vi "Adam_Ch_Input_Output.vi"(0 "Ch names":string[](array[string]), 1 "Previous Scan Value":dbl format="%.2f", 3 "Duty No":u16 format="%016b", 5 "Ch Description":T1={"Ch Name"="", "Type"="", "Function"=enum."Analogue Input", "Ch State"=enum."On", "Calibration type"="", "A"=0.0, "B"=0.0, "C"=0.0, "D"=0.0, "Comments"="", "Address"={"Main"=0, "Ch."=0, "Sub"=0, "Port Name"=""}, "String"="", "Duty"=65535} {"Duty" format="%016b"; "D" format="%#_5g"; "C" format="%#_5g"; "B" format="%#_5g"; "A" format="%#_5g"}, 9 "Scan Period":dbl format="%.2f", 11 "Ch values":dbl[](array[numeric]) format="%.2f", 12 "Value to Output":dbl format="%.2f", 13 "Current Time (sec)":dbl format="%.1f", 14 "Simulate":bool) -> (4 "Calibrated units":dbl format="%_3g", 6 "Good Module":string, 8 "chTime(s)":dbl format="%#_3ps", 10 "Error Row":string[](array[string]), 15 "Scan comment":string)   [LabVIEW 2021]
uses:
  ADAM Client/Sub VIs/ADAM Controls/Ch_description_ADAM.ctl
  ADAM Client/Sub VIs/ADAM Controls/Module_type_ADAM.ctl
  ADAM Client/Sub VIs/ADAM Controls/Function_ADAM.ctl
  ADAM Client/Sub VIs/ADAM Controls/Channel_State.ctl
  ADAM Client/Sub VIs/ADAM Controls/Calib_type_ADAM.ctl
  ADAM Client/Sub VIs/ADAM Controls/Address.ctl
  ADAM_Global.vi
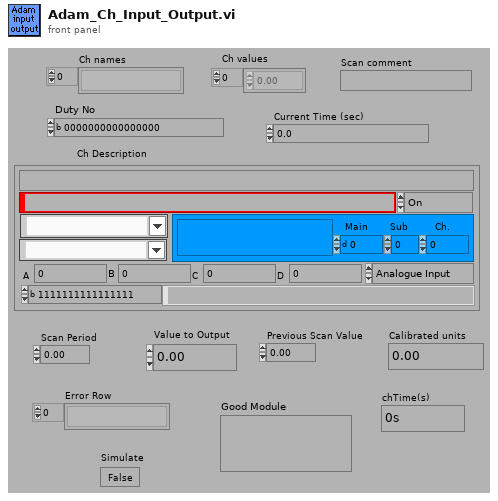
[diagram p1: front panel]
types:
  T1 = typedef "Ch_description_ADAM.ctl" = cluster{"Ch Name":string, "Type":T2, "Function":T3, "Ch State":T4, "Calibration type":T5, "A":dbl, "B":dbl, "C":dbl, "D":dbl, "Comments":string, "Address":T6, "String":string, "Duty":u16}
  T2 = typedef "Module_type_ADAM.ctl" = string
  T3 = typedef "Function_ADAM.ctl" = enum16{"Analogue Input", "Digital Input", "Event counter", "Event rate", "Analogue Output", "Digital Output", "Relay Output"}
  T4 = typedef "Channel_State.ctl" = enum16{"On", "Off", "Always On", "Always Off"}
  T5 = typedef "Calib_type_ADAM.ctl" = string
  T6 = typedef "Address.ctl" = cluster{"Main":i32, "Ch.":i32, "Sub":i32, "Port Name":string}
  T7 = enum16{"On", "Off", "Always On", "Always Off", "Delete"}
  T8 = cluster{"Channel Names":string[], "Last Updated":dbl[]}
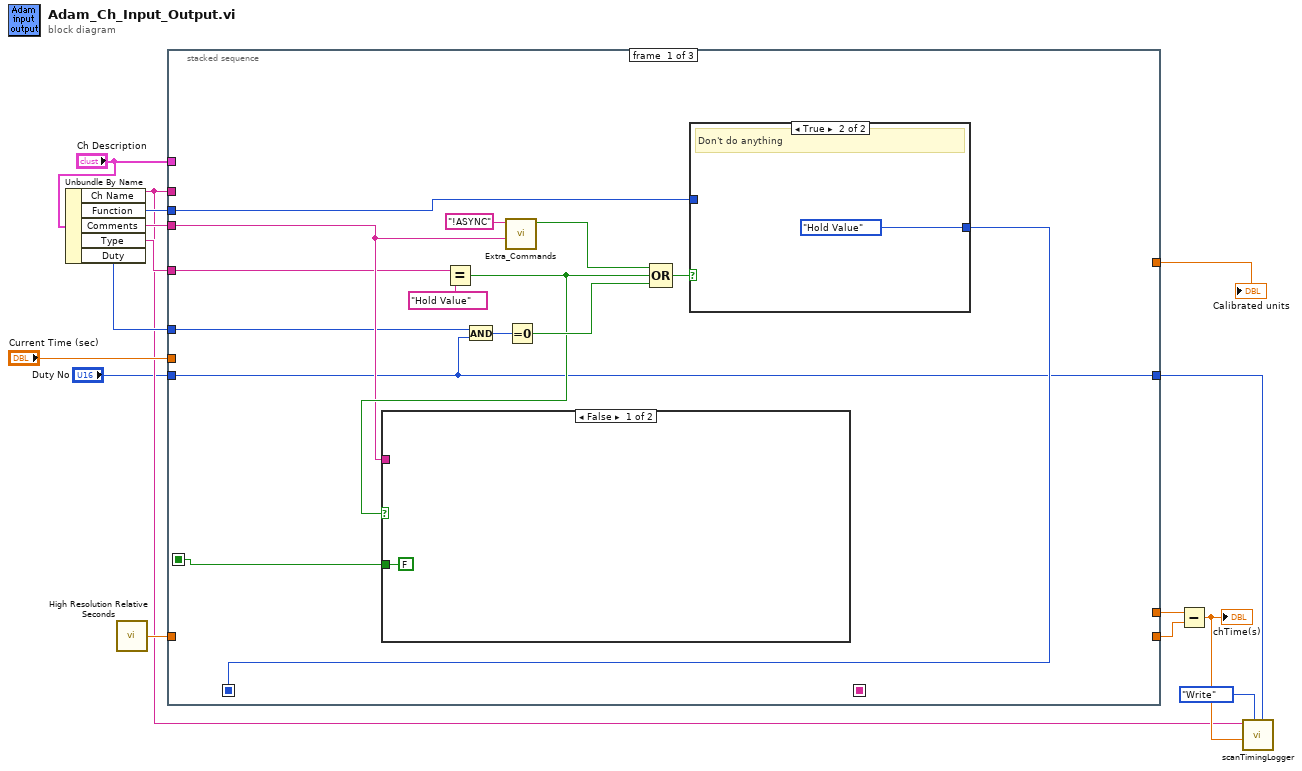
[diagram p0: block diagram]
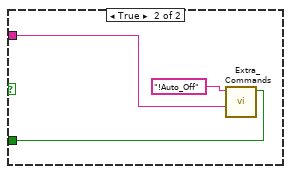
[diagram p2: hidden frame]
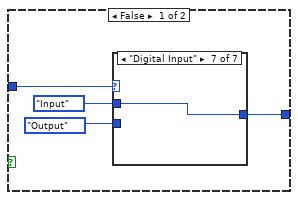
[diagram p3: hidden frame]
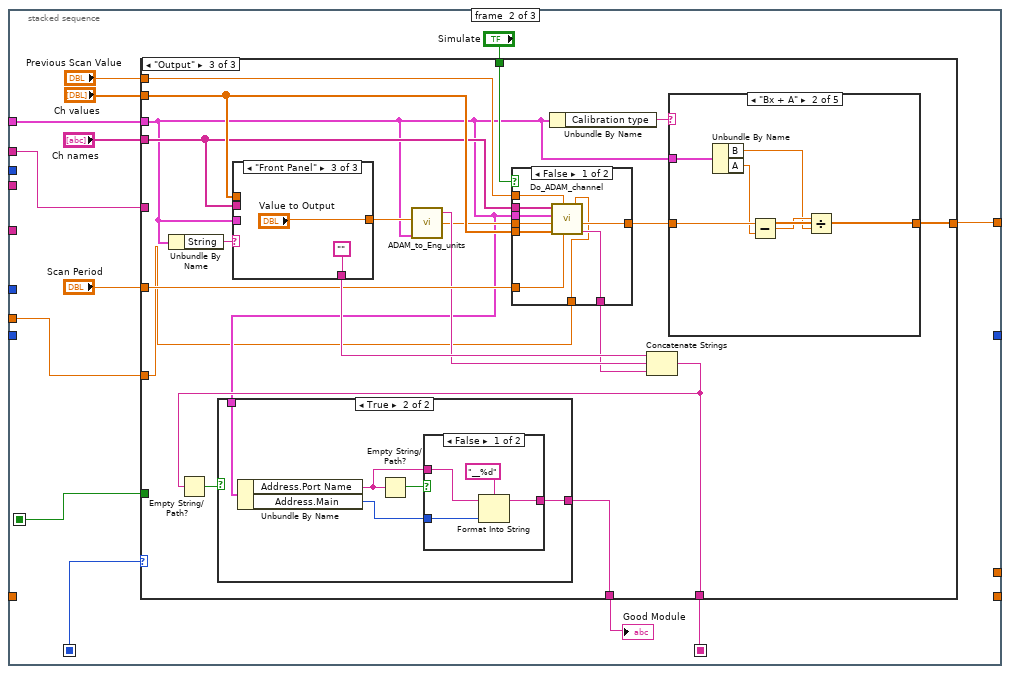
[diagram p10: hidden frame]
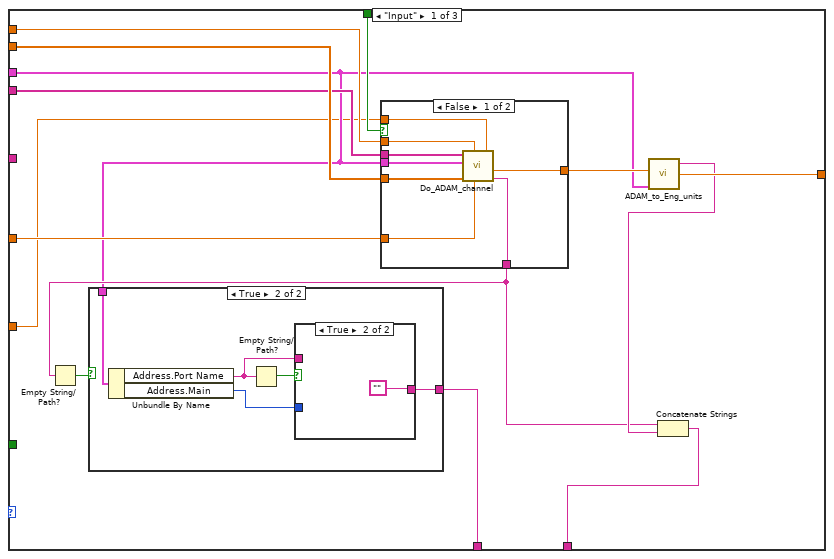
[diagram p11: hidden frame]
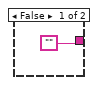
[diagram p12: hidden frame]
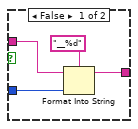
[diagram p13: hidden frame]
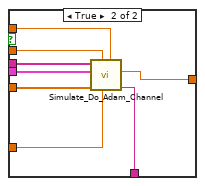
[diagram p14: hidden frame]
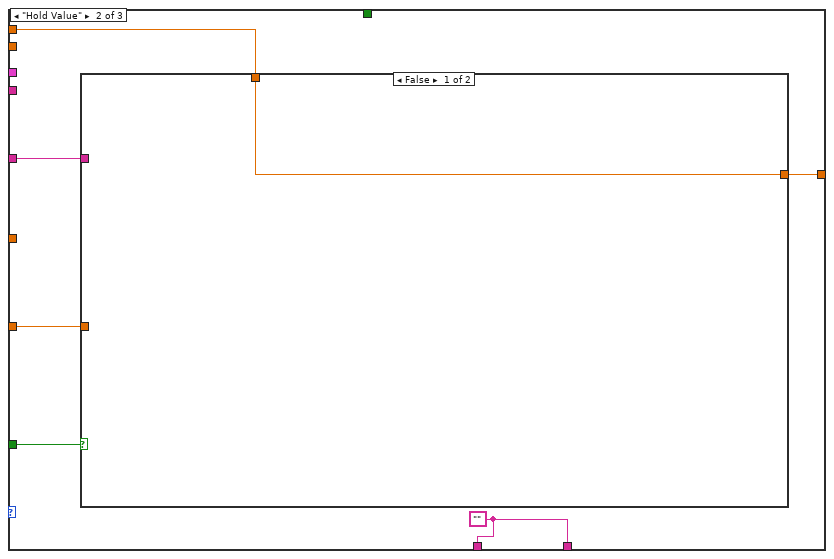
[diagram p15: hidden frame]
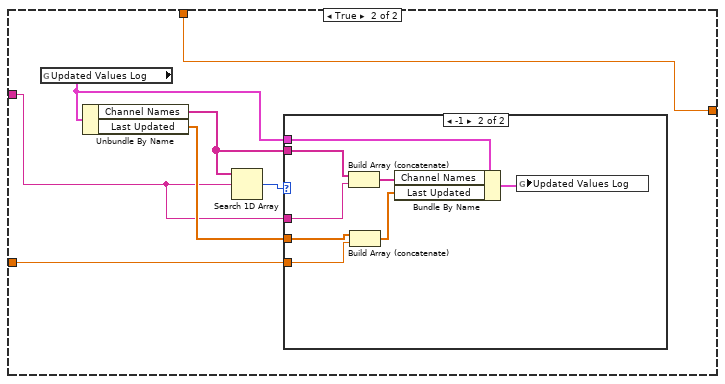
[diagram p16: hidden frame]
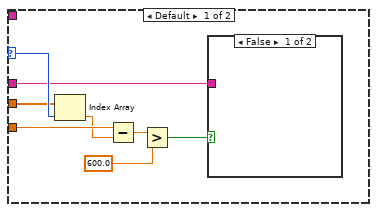
[diagram p17: hidden frame]
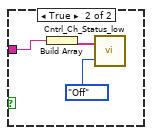
[diagram p18: hidden frame]
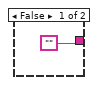
[diagram p19: hidden frame]
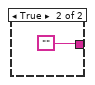
[diagram p20: hidden frame]
diagram:
  n1 = Unbundle By Name("Ch Description") -> ("Ch Name"=w4:string, "Function"=w12:T3, "Comments"=w11:string, "Type"=w10:T2, "Duty"=w9:u16)
  n2 = call <vilib>:"High Resolution Relative Seconds.vi"() -> ("relative seconds"=w6:dbl)
  n3 = stacked-sequence {
    seq-local: [w28 _ _] -> [_ w54 _]
    seq-local: [_ w53 _] -> [_ _ w225]
    seq-local: [w21 _ _] -> [_ w48 _]
    tunnel: "Ch Description" -> [_ w56 w224]
    tunnel: [_ w50 _] -> w14
    tunnel: "Current Time (sec)" -> [_ w47 _]
    tunnel: w12 -> [w20 _ _]
    tunnel: w11 -> [w19 _ _]
    tunnel: w10 -> [w18 _ _]
    tunnel: w9 -> [w17 _ _]
    tunnel: w4 -> [_ w46 _]
    tunnel: [_ _ w222] -> w8
    tunnel: [_ _ w221] -> w7
    tunnel: w6 -> [_ _ w221]
    tunnel: [w16 _ _] -> w2
    tunnel: "Duty No" -> [w16 _ _]
    frame #0 {
      n4 = Equal?(x=w18, y=T2 "Hold Value" ("Type")) -> (x = y?=w22:bool)
      n5 = case shown="False" w22 {
        tunnel: w19 -> [_ w33]
        tunnel: [FALSE ("Command Found") w31] -> w21
        frame False {
        }
        frame True {
          n6 = call "Extra_Commands.vi"("String to Search"=w33, "Command"="!Auto_Off" ("String to match")) -> ("Command Found"=w31:bool)  [unwired: 1 in, 4 out]
        }
      }
      n7 = And(x=w17, y=w16) -> (x .and. y?=w25:u16)
      n8 = call "Extra_Commands.vi"("String to Search"=w19, "Command"="!ASYNC" ("String to match")) -> ("Command Found"=w26:bool)  [unwired: 1 in, 4 out]
      n9 = Equal To 0?(x=w25) -> (x = 0?=w24:bool)
      n10 = Compound Arithmetic op=OR(w26, w22, w24) -> (w23:bool)
      n11 = case shown="True" w23 {
        tunnel: w20 -> [w35 _]
        tunnel: [w34 enum16{"Input", "Output", "Hold Value"}."Hold Value"] -> w28
        frame False {
          n12 = case shown="\"Digital Input\"" w35 {
            tunnel: [w38 w39 w40 w41 w42 w43 w44] -> w34
            tunnel: enum16{"Input", "Output", "Hold Value"}."Input" -> [w38 w39 w40 _ _ _ w44]
            tunnel: enum16{"Input", "Output", "Hold Value"}."Output" -> [_ _ _ w41 w42 w43 _]
            frame "Analogue Input" {
            }
            frame "Event counter" {
            }
            frame "Event rate" {
            }
            frame "Analogue Output" {
            }
            frame "Digital Output" {
            }
            frame "Relay Output" {
            }
            frame "Digital Input" {
            }
          }
        }
        frame True {
          # "Don't do anything"
        }
      }
    }
    frame #1 {
      n13 = case shown="\"Output\"" w54 {
        tunnel: [w72 w103 w140] -> w50
        tunnel: "Scan Period" -> [w68 _ w145]
        tunnel: "Ch values" -> [w70 _ w151]
        tunnel: "Ch names" -> [w69 _ w150]
        tunnel: [w65 w100 w136] -> w53
        tunnel: w56 -> [w61 _ w134]
        tunnel: "Previous Scan Value" -> [w67 w104 w148]
        tunnel: "Simulate" -> [w64 _ w142]
        tunnel: [w60 w100 w135] -> w49
        tunnel: w48 -> [_ w105 _]
        tunnel: w47 -> [w59 w101 w133]
        tunnel: w46 -> [_ w102 _]
        frame "Input" {
          n14 = case shown="False" w64 {
            tunnel: [w91 w99] -> w71
            tunnel: w70 -> [w90 w98]
            tunnel: w69 -> [w89 w97]
            tunnel: w61 -> [w85 w96]
            tunnel: w68 -> [w88 w95]
            tunnel: w67 -> [w87 w94]
            tunnel: [w86 w93] -> w62
            tunnel: w59 -> [w84 w92]
            frame False {
              n15 = call "Do_ADAM_channel.vi"("Current Time (sec)"=w84, "Scan Period"=w88, "Previous Scan Value"=w87, "Present scan array"=w90, "Ch Description"=w85, "Ch names"=w89) -> ("Scan comment"=w86:string, "Output"=w91:dbl)  [unwired: 1 in, 1 out]
            }
            frame True {
              n16 = call "Simulate_Do_Adam_Channel.vi"("Current Time (sec)"=w92, "Scan Period"=w95, "Previuos Scan Value"=w94, "Ch values"=w98, "Ch Discription"=w96, "Ch names"=w97) -> ("Scan comment"=w93:string, "Calibrated units"=w99:dbl)  [unwired: 3 in]
            }
          }
          n17 = Empty String/Path?(string/path=w62) -> (empty?=w63:bool)
          n18 = case shown="True" w63 {
            tunnel: w61 -> [_ w75]
            tunnel: ["" w74] -> w60
            frame False {
            }
            frame True {
              n19 = Unbundle By Name(w75) -> ("Address.Port Name"=w77:string, "Address.Main"=w76:i32)
              n20 = Empty String/Path?(string/path=w77) -> (empty?=w78:bool)
              n21 = case shown="True" w78 {
                tunnel: w77 -> [w82 _]
                tunnel: w76 -> [w81 _]
                tunnel: [w79 ""] -> w74
                frame False {
                  n22 = Format Into String(format string="__%d", initial string=w82, w81) -> (resulting string=w79:string)  [unwired: 1 in, 1 out]
                }
                frame True {
                }
              }
            }
          }
          n23 = call "ADAM_to_Eng_units.vi"("Ch Description"=w61, "Raw"=w71) -> ("Calibrated units"=w72:dbl, "Comments"=w66:string)  [unwired: 1 in, 2 out]
          n24 = Concatenate Strings(w62, w66) -> (w65:string)
        }
        frame "Hold Value" {
          w100 = ""
          n25 = case shown="False" w105 {
            tunnel: w104 -> [w106 w110]
            tunnel: [w106 w110] -> w103
            tunnel: w102 -> [_ w107]
            tunnel: w101 -> [_ w111]
            frame False {
            }
            frame True {
              n26 = global read "ADAM_Global.vi" "Updated Values Log"() -> (w109:T8)
              n27 = Unbundle By Name(w109) -> ("Channel Names"=w108:string[], "Last Updated"=w112:dbl[])
              n28 = Search 1D Array(1D array=w108, element=w107) -> (index of element=w113:i32)  [unwired: 1 out]
              n29 = case shown="-1" w113 {
                selector: w113 -> [w121 _]
                tunnel: w112 -> [w120 w128]
                tunnel: w111 -> [w119 w127]
                tunnel: w109 -> [_ w132]
                tunnel: w108 -> [_ w131]
                tunnel: w107 -> [w114 w129]
                frame Default {
                  n30 = Index Array(array=w120, index=w121) -> (element=w118:dbl)
                  n31 = Subtract(x=w119, y=w118) -> (x-y=w117:dbl)
                  n32 = Greater?(x=w117, y=600.0) -> (0:w115:bool)
                  n33 = case shown="False" w115 {
                    tunnel: w114 -> [_ w122]
                    frame False {
                    }
                    frame True {
                      n34 = Build Array(w122) -> (w123:string[])
                      n35 = call "Cntrl_Ch_Status_low.vi"("Mode"=T7."Off", "Channel names"=w123) -> ()  [unwired: 1 out]
                    }
                  }
                }
                frame -1 {
                  n36 = Build Array (concatenate)(w131, w129) -> (w130:string[])
                  n37 = Build Array (concatenate)(w128, w127) -> (w126:dbl[])
                  n38 = Bundle By Name(cluster=w132, "Channel Names"=w130, "Last Updated"=w126) -> (w125:T8)
                  n39 = global write "ADAM_Global.vi" "Updated Values Log"(w125) -> ()
                }
              }
            }
          }
        }
        frame "Output" {
          n40 = Unbundle By Name(w134) -> ("String"=w147:string)
          n41 = case shown="\"Front Panel\"" w147 {
            selector: w147 -> [w211 _ _]
            tunnel: w134 -> [_ w218 _]
            tunnel: w151 -> [w215 _ _]
            tunnel: w150 -> [w214 _ _]
            tunnel: [w213 "" ""] -> w149
            tunnel: [w212 w216 "Value to Output"] -> w146
            frame "Other", Default {
              n42 = call "Read_value_of_earlier_Ch.vi"("Desired Ch to Read"=w211, "Ch names"=w214, "Present scan array"=w215) -> ("Value"=w212:dbl, "Scan comment"=w213:string)  [unwired: 1 in]
            }
            frame "Read A" {
              n43 = Unbundle By Name(w218) -> ("A"=w216:dbl)
            }
            frame "Front Panel" {
            }
          }
          n44 = call "ADAM_to_Eng_units.vi"("Ch Description"=w134, "Raw"=w146) -> ("Calibrated units"=w143:dbl, "Comments"=w144:string)  [unwired: 1 in, 2 out]
          n45 = case shown="False" w142 {
            tunnel: w151 -> [w201 w210]
            tunnel: w150 -> [w200 w209]
            tunnel: [w199 w208] -> w139
            tunnel: w148 -> [w198 w207]
            tunnel: [w197 w206] -> w138
            tunnel: w145 -> [w196 w205]
            tunnel: w134 -> [w195 w204]
            tunnel: w143 -> [w194 w203]
            tunnel: w133 -> [w193 w202]
            frame False {
              n46 = call "Do_ADAM_channel.vi"("Current Time (sec)"=w193, "Scan Period"=w196, "Previous Scan Value"=w198, "Present scan array"=w201, "Value to Output"=w194, "Ch Description"=w195, "Ch names"=w200) -> ("Scan comment"=w197:string, "Output"=w199:dbl)  [unwired: 1 out]
            }
            frame True {
              n47 = call "Simulate_Do_Adam_Channel.vi"("Current Time (sec)"=w202, "Scan Period"=w205, "Previuos Scan Value"=w207, "Ch values"=w210, "Value to Output"=w203, "Ch Discription"=w204, "Ch names"=w209) -> ("Scan comment"=w206:string, "Calibrated units"=w208:dbl)  [unwired: 2 in]
            }
          }
          n48 = Unbundle By Name(w134) -> ("Calibration type"=w141:T5)
          n49 = Concatenate Strings(w149, w144, w138) -> (w136:string)
          n50 = Empty String/Path?(string/path=w136) -> (empty?=w137:bool)
          n51 = case shown="True" w137 {
            tunnel: w134 -> [_ w154]
            tunnel: ["" w153] -> w135
            frame False {
            }
            frame True {
              n52 = Unbundle By Name(w154) -> ("Address.Port Name"=w156:string, "Address.Main"=w155:i32)
              n53 = Empty String/Path?(string/path=w156) -> (empty?=w157:bool)
              n54 = case shown="False" w157 {
                tunnel: w156 -> [w161 _]
                tunnel: w155 -> [w160 _]
                tunnel: [w158 ""] -> w153
                frame False {
                  n55 = Format Into String(format string="__%d", initial string=w161, w160) -> (resulting string=w158:string)  [unwired: 1 in, 1 out]
                }
                frame True {
                }
              }
            }
          }
          n56 = case shown="\"Bx + A\"" w141 {
            tunnel: [w163 w165 w170 w178 w186] -> w140
            tunnel: w139 -> [w163 w168 w171 w179 w189]
            tunnel: w134 -> [_ w169 w176 w184 w192]
            frame "Raw", Default {
            }
            frame "Bx + A" {
              n57 = Unbundle By Name(w169) -> ("B"=w164:dbl, "A"=w167:dbl)
              n58 = Subtract(x=w168, y=w167) -> (x-y=w166:dbl)
              n59 = Divide(x=w166, y=w164) -> (x/y=w165:dbl)
            }
            frame "Cx^2 + Bx + A" {
              n60 = Unbundle By Name(w176) -> ("A"=w175:dbl, "B"=w174:dbl, "C"=w173:dbl)
              n61 = Build Array(w175, w174, w173) -> (w172:dbl[])
              n62 = call "Polybackwards.vi"("Coefficients"=w172, "Y input"=w171) -> ("X output"=w170:dbl)  [unwired: 1 out]
            }
            frame "Dx^3 + Cx^2 + Bx + A" {
              n63 = Unbundle By Name(w184) -> ("A"=w183:dbl, "B"=w182:dbl, "C"=w181:dbl, "D"=w177:dbl)
              n64 = Build Array(w183, w182, w181, w177) -> (w180:dbl[])
              n65 = call "Polybackwards.vi"("Coefficients"=w180, "Y input"=w179) -> ("X output"=w178:dbl)  [unwired: 1 out]
            }
            frame "Cropped Amin Bmax" {
              n66 = Unbundle By Name(w192) -> ("A"=w191:dbl, "B"=w190:dbl)
              n67 = In Range and Coerce(upper limit=w191, x=w189, lower limit=w190) -> (coerced(x)=w187:dbl, In Range?=w188:bool)
              n68 = Select(t=w187, s=w188, f=nan) -> (s? t:f=w186:dbl)
            }
          }
        }
      }
      "Good Module" <- w49
    }
    frame #2 {
      n69 = Empty String/Path?(string/path=w225) -> (empty?=w226:bool)
      n70 = case shown="False" w226 {
        tunnel: w225 -> [w229 w244]
        tunnel: [w239 w244] -> w227
        tunnel: w224 -> [w238 _]
        tunnel: [w228 string[] []] -> w223
        frame False {
          n71 = Unbundle By Name(w238) -> ("Ch Name"=w237:string, "Address.Port Name"=w236:string, "Address.Main"=w235:i32, "Address.Sub"=w233:i32, "Type"=w231:T2)
          n72 = Concatenate Strings(w231) -> (w230:string)
          n73 = Number To Decimal String(number=w235) -> (decimal integer string=w234:string)  [unwired: 1 in]
          n74 = Number To Decimal String(number=w233) -> (decimal integer string=w232:string)  [unwired: 1 in]
          n75 = Concatenate Strings("(", w237, ":" ("Scan comment"), w229, ")") -> (w239:string)
          n76 = Build Array(w237, w236, w234, w232, w230, w229) -> (w228:string[])
        }
        frame True {
        }
      }
      "Scan comment" <- w227
      "Error Row" <- w223
      n77 = call <vilib>:"High Resolution Relative Seconds.vi"() -> ("relative seconds"=w222:dbl)
    }
  }
  "Calibrated units" <- w14
  n78 = Subtract(x=w8, y=w7) -> (x-y=w5:dbl)
  "chTime(s)" <- w5
  n79 = call "scanTimingLogger.vi"("duty"=w2, "mode"=enum16{"Write", "Read", "Flush"}."Write", "time"=w5, "name"=w4) -> ()  [unwired: 6 in, 2 out]
